vi "video.create_add_label.vi"(8 "error in":errorcluster, 11 "VideoCreateStaging in":refnum<class "VideoCreateStaging.lvclass">) -> (0 "error out":errorcluster, 3 "VideoCreateStaging out":refnum<class "VideoCreateStaging.lvclass">)   [LabVIEW 2020, in "VideoCreateStaging.lvclass"]
doc: "Adds a label to the video being created."
uses:
  VideoCreateStaging.lvclass
  VideoCreateStaging.lvclass/VideoCreateStaging.ctl
  client.lvlib
panel:
  in  "label":string
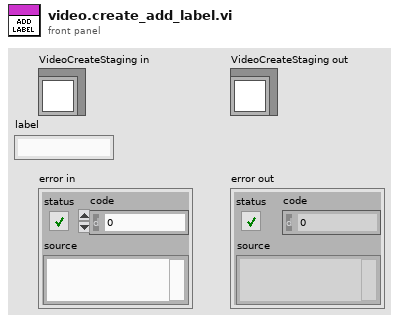
[diagram p1: front panel]
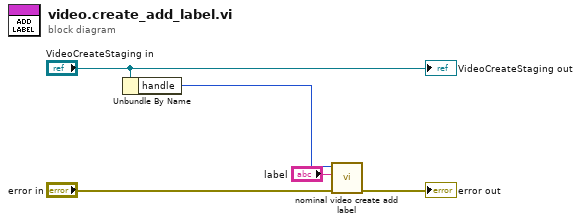
[diagram p0: block diagram]
diagram:
  n1 = Unbundle By Name("VideoCreateStaging in") -> ("handle"=w3:i32)
  n2 = call "nominal video create add label.vi"("error in (no error)"="error in", "label"="label", "staging"=w3) -> ("error out"=→"error out":errorcluster)  [unwired: 7 in, 1 out]
  "VideoCreateStaging out" <- "VideoCreateStaging in"
